vi "InfoGui.vi"(10 "_Msg":string) -> (2 "ok":bool)   [LabVIEW 2019, in "Tools.lvlib"]
uses:
  Tools.lvlib
  controls/buttons/OK.ctl
  controls/buttons/Cancel.ctl
  InfoGui.Action.ctl
panel:
  out "_loop":i32(ring)=4
  in  "open?":bool
  in  "CancelButton":T1
  out "Message":string
  in  "OKButton":T2
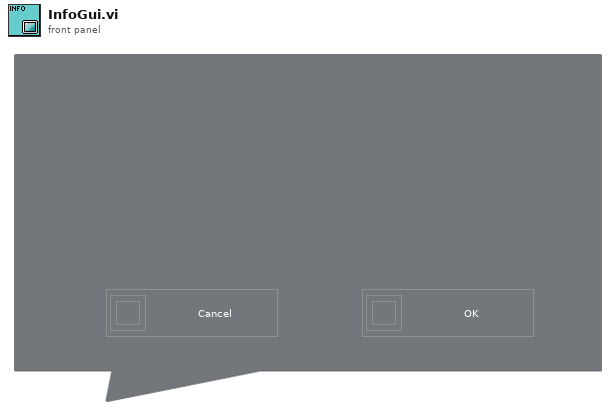
[diagram p1: front panel]
types:
  T1 = typedef "Tools.lvlib/Cancel.ctl" = bool
  T2 = typedef "Tools.lvlib/OK.ctl" = bool
  T3 = typedef "Tools.lvlib/InfoGui.Action.ctl" = enum32{"idle", "constructor", "destructor", "--- InfoGUI ---", "Gui.Translate"}
  T4 = enum32{"invalid app kind", "Development System", "Run Time System", "Student Edition", "Embedded LabVIEW", "Evaluation", "Custom"}
  T5 = typedef "LVPositionTypeDef.ctl" = cluster{"Left":i32, "Top":i32}
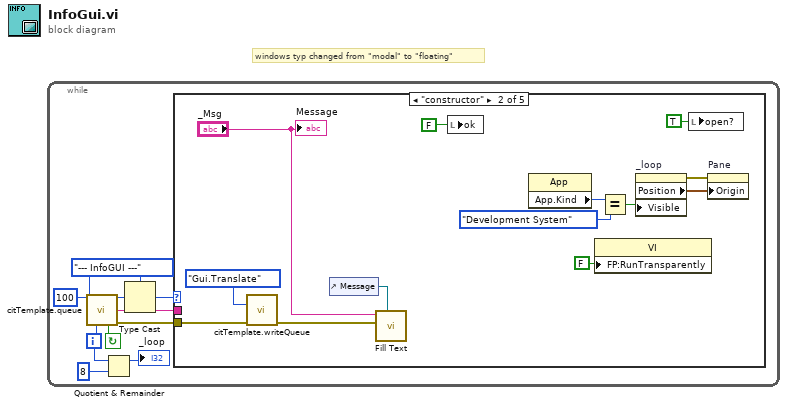
[diagram p0: block diagram]
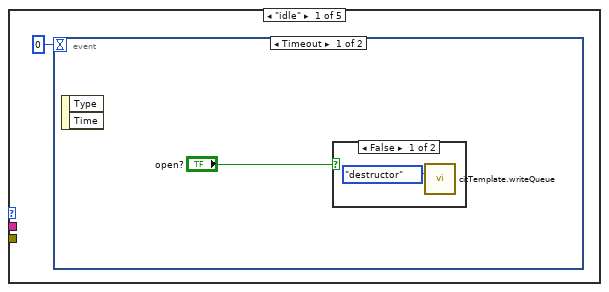
[diagram p2: hidden frame]
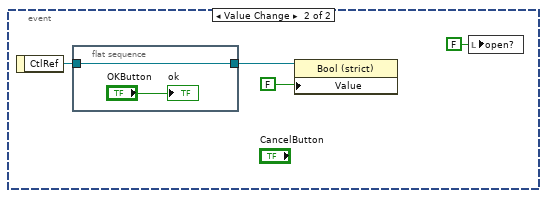
[diagram p4: hidden frame]
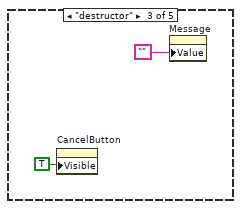
[diagram p5: hidden frame]
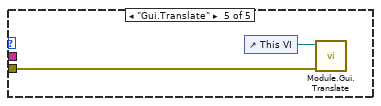
[diagram p7: hidden frame]
diagram:
  # "windows typ changed from \"modal\" to \"floating\""
  n1 = while {
    i -> [w1]
    stop <- w10 continue-if-true
    w4 = InfoGui.Action."--- InfoGUI ---" ("Action")
    n2 = call "citTemplate.queue.vi"("ms timeout (250 ms)"=100, "event enum"=w4, "iteration (-1)"=w1) -> ("event out"=w8:u32, "(flatten) data out"=w5:string, "continue"=w10:bool, "error out"=w6:errorcluster)  [unwired: 2 in, 7 out]
    n3 = Quotient & Remainder(x=w1, y=8) -> (x-y*floor(x/y)=→"_loop":i32)  [unwired: 1 out]
    n4 = Type Cast(type=w4, x=w8) -> (*(type *) &x=w7:T3)
    n5 = case shown="\"constructor\"" w7 {
      tunnel: w6 -> [_ w24 _ _ w35]
      tunnel: w5 -> [_ _ _ _ _]
      frame "idle" {
        n6 = event shown="[0] Timeout" {
          selector: _ -> [_ _]
          dyn-events: _ -> [_ _]
          timeout: 0 -> [_ _]
          event Timeout {
            n7 = event-data() -> ()  [unwired: 3 out]
            n8 = case shown="False" "open?" {
              frame False {
                n9 = call "citTemplate.writeQueue.vi"("event in (if not connected:all statemachine with data event)"=InfoGui.Action."destructor" ("Action")) -> ()  [unwired: 4 in, 11 out]
              }
              frame True {
              }
            }
          }
          event Value Change {
            n10 = event-data() -> ("CtlRef"=w16:refnum<vi>)  [unwired: 1 out]
            n11 = flat-sequence {
              tunnel: w16 -> [w18]
              tunnel: [w18] -> w15
              frame #0 {
                "ok" <- "OKButton"
              }
            }
            n12 = property class="Bool (strict)"(reference=w15, "Value"=T2 FALSE) -> ()  [unwired: 1 in, 2 out]
            n13 = local write "open?"(FALSE ("open?")) -> ()
          }
        }
      }
      frame "constructor" {
        n14 = call "citTemplate.writeQueue.vi"("event in (if not connected:all statemachine with data event)"=InfoGui.Action."Gui.Translate" ("Action"), "error in (no error)"=w24) -> ("error out"=w22:errorcluster)  [unwired: 13 in]
        n15 = control-ref of="Message"() -> (w21:refnum<vi>)
        n16 = call "Fill Text.vi"("String ref"=w21, "Error In"=w22, "String in"="_Msg") -> ()  [unwired: 8 in, 1 out]
        n17 = local write "ok"(FALSE ("_b_ok")) -> ()
        n18 = property class="App"() -> ("App.Kind"=w27:T4)  [unwired: 2 in, 2 out]
        n19 = property class="VI"("FP:RunTransparently"=FALSE ("Front Panel Window:Run VI Transparently")) -> ()  [unwired: 2 in, 2 out]
        n20 = Equal?(x=w27, y=T4."Development System") -> (x = y?=w25:bool)
        n21 = property on="_loop" class="Ring (strict)"("Visible"=w25) -> (error out=w28:errorcluster, "Position"=w29:T5)  [unwired: 2 in, 1 out]
        n22 = local write "open?"(TRUE ("open?")) -> ()
        n23 = property on="Pane" class="Pane"(error in=w28, "Origin"=w29) -> ()  [unwired: 1 in, 2 out]
        "Message" <- "_Msg"
      }
      frame "destructor" {
        n24 = property on="CancelButton" class="Bool (strict)"("Visible"=TRUE) -> ()  [unwired: 2 in, 2 out]
        n25 = property on="Message" class="Str"("Value"="") -> ()  [unwired: 2 in, 2 out]
      }
      frame "--- InfoGUI ---" {
      }
      frame "Gui.Translate" {
        n26 = control-ref of="This VI"() -> (w36:refnum<vi>)
        n27 = call "Module.Gui.Translate.vi"("error in"=w35, "VI ref in"=w36) -> ()  [unwired: 7 in, 3 out]
      }
    }
  }
